vi "Doe_Julabo_Control_subVI_2.vi"(0 "Julabo CF41 VISA":refnum<visa-resource-name>="COM3", 1 "Data Cluster In":T1={"Current DoE"=[], "SSI 1 Flow Rate"=0.0, "SSI 2 Flow Rate"=0.0, "FLOM 1 Flow Rate"=0.0, "FLOM 2 Flow Rate"=0.0, "Pumps Running?"=FALSE, "Boolean 2"=FALSE, "Boolean 3"=FALSE, "Boolean 4"=FALSE, "At Equilibrium?"=FALSE, "Script Running?"=FALSE, "Current Script Iteration"=0.0, "Total Script Iterations"=0.0, "FLOM Pumps VISA"="COM2", "SSI 1 Pump VISA"="COM76", "SSI 2 Pump VISA"="COM74", "Huber Unistat VISA"="COM1", "SSI 3 Pump VISA"="COM76", "SSI 4 Pump VISA"="COM76", "SSI 4 Flow Rate"=0.0, "SSI 3 Flow Rate"=0.0, "Flow Meter 1 Rate "=0.0, "Flow Meter 2 Rate"=0.0, "Flow Meter 3 Rate"=0.0, "Flow Meter 4 Rate"=0.0, "SSI 1 Flow Setpoint"=0.0, "SSI 2 Flow Setpoint"=0.0, "SSI 3 Flow Setpoint"=0.0, "SSI 4 Flow Setpoint"=0.0, "Temperature Setpoint"=0.0, "Flow meter 3 COM"=17, "Flow meter 5 COM"=18, "Flow meter 4 COM"=19, "Flow meter 2 COM"=16, "Flow meter 1 COM"=15, "Unit"=enum."PSI", "Pressure COM"="COM6", "Julabo Setpoint"=0.0, "Julabo Control"=enum."Internal", "Overtemp"=50.0, "Subtemp"=-20.0, "HeatMax"=50, "CoolMax"=-100, "InternMax"=50.0, "InternMin"=0.0, "Upper Bandlimit"=100.0, "Lower Bandlimit"=0.0, "Julabo CF41 VISA"="COM3", "Xp (0.6K) Int"=0.6, "Tn (3s) Int"=3, "Tv (0s) Int"=0, "Dynamic (0: aperiodic) Int"=enum."aperiodic", "Xp (0.6K) Ext"=0.6, "Tn (3s) Ext"=3, "Tv (0s) Ext"=0, "XpU (0.6K) Ext"=0.6, "Julabo Serial Configuration"={"Baud Rate"=4800, "Parity"=2, "Data Bits"=7, "Stop Bits"=10, "Flow Control"=2}} {"Julabo Serial Configuration"."Flow Control" items=["None", "XON/XOFF", "RTS/CTS", "XON/XOFF & RTS/CTS", "DTR/DSR", "XON/XOFF & DTR/DSR"]; "Julabo Serial Configuration"."Stop Bits" items=["1.0"=10, "1.5"=15, "2.0"=20]; "Julabo Serial Configuration"."Data Bits" items=["7"=7, "8"=8]; "Julabo Serial Configuration"."Parity" items=["None", "Odd", "Even", "Mark", "Space"]; "Julabo Serial Configuration"."Baud Rate" items=["300"=300, "600"=600, "1200"=1200, "2400"=2400, "4800"=4800, "9600"=9600, "19200"=19200]; "XpU (0.6K) Ext" min=0.1 max=99.9; "Tv (0s) Ext" max=999; "Tn (3s) Ext" min=3 max=9999; "Xp (0.6K) Ext" min=0.1 max=99.9; "Tv (0s) Int" max=999; "Tn (3s) Int" min=3 max=9999; "Xp (0.6K) Int" min=0.1 max=99.9; "Lower Bandlimit" min=0.0 max=200.0; "Upper Bandlimit" min=0.0 max=200.0; "InternMin" format="%.2f"; "InternMax" format="%.2f"; "CoolMax" min=-100 max=0; "HeatMax" max=100; "Subtemp" format="%.2f"; "Overtemp" format="%.2f"; "Julabo Setpoint" format="%.2f"; "Current DoE" format="%0.3f"}, 2 "Case Selector":string, 3 "StartStop":bool) -> (4 "Data Cluster Out":T1={"Current DoE"=[], "SSI 1 Flow Rate"=0.0, "SSI 2 Flow Rate"=0.0, "FLOM 1 Flow Rate"=0.0, "FLOM 2 Flow Rate"=0.0, "Pumps Running?"=FALSE, "Boolean 2"=FALSE, "Boolean 3"=FALSE, "Boolean 4"=FALSE, "At Equilibrium?"=FALSE, "Script Running?"=FALSE, "Current Script Iteration"=0.0, "Total Script Iterations"=0.0, "FLOM Pumps VISA"="COM2", "SSI 1 Pump VISA"="COM76", "SSI 2 Pump VISA"="COM74", "Huber Unistat VISA"="COM1", "SSI 3 Pump VISA"="COM76", "SSI 4 Pump VISA"="COM76", "SSI 4 Flow Rate"=0.0, "SSI 3 Flow Rate"=0.0, "Flow Meter 1 Rate "=0.0, "Flow Meter 2 Rate"=0.0, "Flow Meter 3 Rate"=0.0, "Flow Meter 4 Rate"=0.0, "SSI 1 Flow Setpoint"=0.0, "SSI 2 Flow Setpoint"=0.0, "SSI 3 Flow Setpoint"=0.0, "SSI 4 Flow Setpoint"=0.0, "Temperature Setpoint"=0.0, "Flow meter 3 COM"=17, "Flow meter 5 COM"=18, "Flow meter 4 COM"=19, "Flow meter 2 COM"=16, "Flow meter 1 COM"=15, "Unit"=enum."PSI", "Pressure COM"="COM6", "Julabo Setpoint"=0.0, "Julabo Control"=enum."Internal", "Overtemp"=50.0, "Subtemp"=-20.0, "HeatMax"=50, "CoolMax"=-100, "InternMax"=50.0, "InternMin"=0.0, "Upper Bandlimit"=100.0, "Lower Bandlimit"=0.0, "Julabo CF41 VISA"="COM3", "Xp (0.6K) Int"=0.6, "Tn (3s) Int"=3, "Tv (0s) Int"=0, "Dynamic (0: aperiodic) Int"=enum."aperiodic", "Xp (0.6K) Ext"=0.6, "Tn (3s) Ext"=3, "Tv (0s) Ext"=0, "XpU (0.6K) Ext"=0.6, "Julabo Serial Configuration"={"Baud Rate"=4800, "Parity"=2, "Data Bits"=7, "Stop Bits"=10, "Flow Control"=2}} {"Julabo Serial Configuration"."Flow Control" items=["None", "XON/XOFF", "RTS/CTS", "XON/XOFF & RTS/CTS", "DTR/DSR", "XON/XOFF & DTR/DSR"]; "Julabo Serial Configuration"."Stop Bits" items=["1.0"=10, "1.5"=15, "2.0"=20]; "Julabo Serial Configuration"."Data Bits" items=["7"=7, "8"=8]; "Julabo Serial Configuration"."Parity" items=["None", "Odd", "Even", "Mark", "Space"]; "Julabo Serial Configuration"."Baud Rate" items=["300"=300, "600"=600, "1200"=1200, "2400"=2400, "4800"=4800, "9600"=9600, "19200"=19200]; "XpU (0.6K) Ext" min=0.1 max=99.9; "Tv (0s) Ext" max=999; "Tn (3s) Ext" min=3 max=9999; "Xp (0.6K) Ext" min=0.1 max=99.9; "Tv (0s) Int" max=999; "Tn (3s) Int" min=3 max=9999; "Xp (0.6K) Int" min=0.1 max=99.9; "Lower Bandlimit" min=0.0 max=200.0; "Upper Bandlimit" min=0.0 max=200.0; "InternMin" format="%.2f"; "InternMax" format="%.2f"; "CoolMax" min=-100 max=0; "HeatMax" max=100; "Subtemp" format="%.2f"; "Overtemp" format="%.2f"; "Julabo Setpoint" format="%.2f"; "Current DoE" format="%0.3f"}, 15 "error out 2":errorcluster caption="error out")   [LabVIEW 2015, in "JULABO DeviceDriver.lvlib"]
doc: "Advanced event triggered example"
uses:
  <instrlib>/JULABO DeviceDriver/JULABO DeviceDriver.lvlib
  --Controls and TypeDefs--/DoE_Control_Cluster.ctl
  <instrlib>/JULABO DeviceDriver/Examples/Julabo Serial Control.ctl
panel:
  in  "error in":errorcluster
  out "device error out":errorcluster
  in  "Setpointindex":enum16{"Setpoint 1", "Setpoint 2", "Setpoint 3"}(ring)
  in  "Registerkartenelement":T3(tab)
  # "Note: Julabo must be set to Set Temp - RS232\nfor commands to properly write to unit!!!!!"
  # "1. Select the COM-Port and adjust the serial\nconfiguration for your instrument\n2. Adjust the Read cycle\n3. Start the VI by pressing the \"Start\" -Button\n( Arrow button on the top-left corner)\n4. To stop the execution press the \"Stop\" button"
  # "Julabo"
  # "Limits"
  # "PID Control Parameters"
  # "Julabo"
  # "Limits"
  # "PID Control Parameters"
  # "Internal parameters"
  # "External parameters"
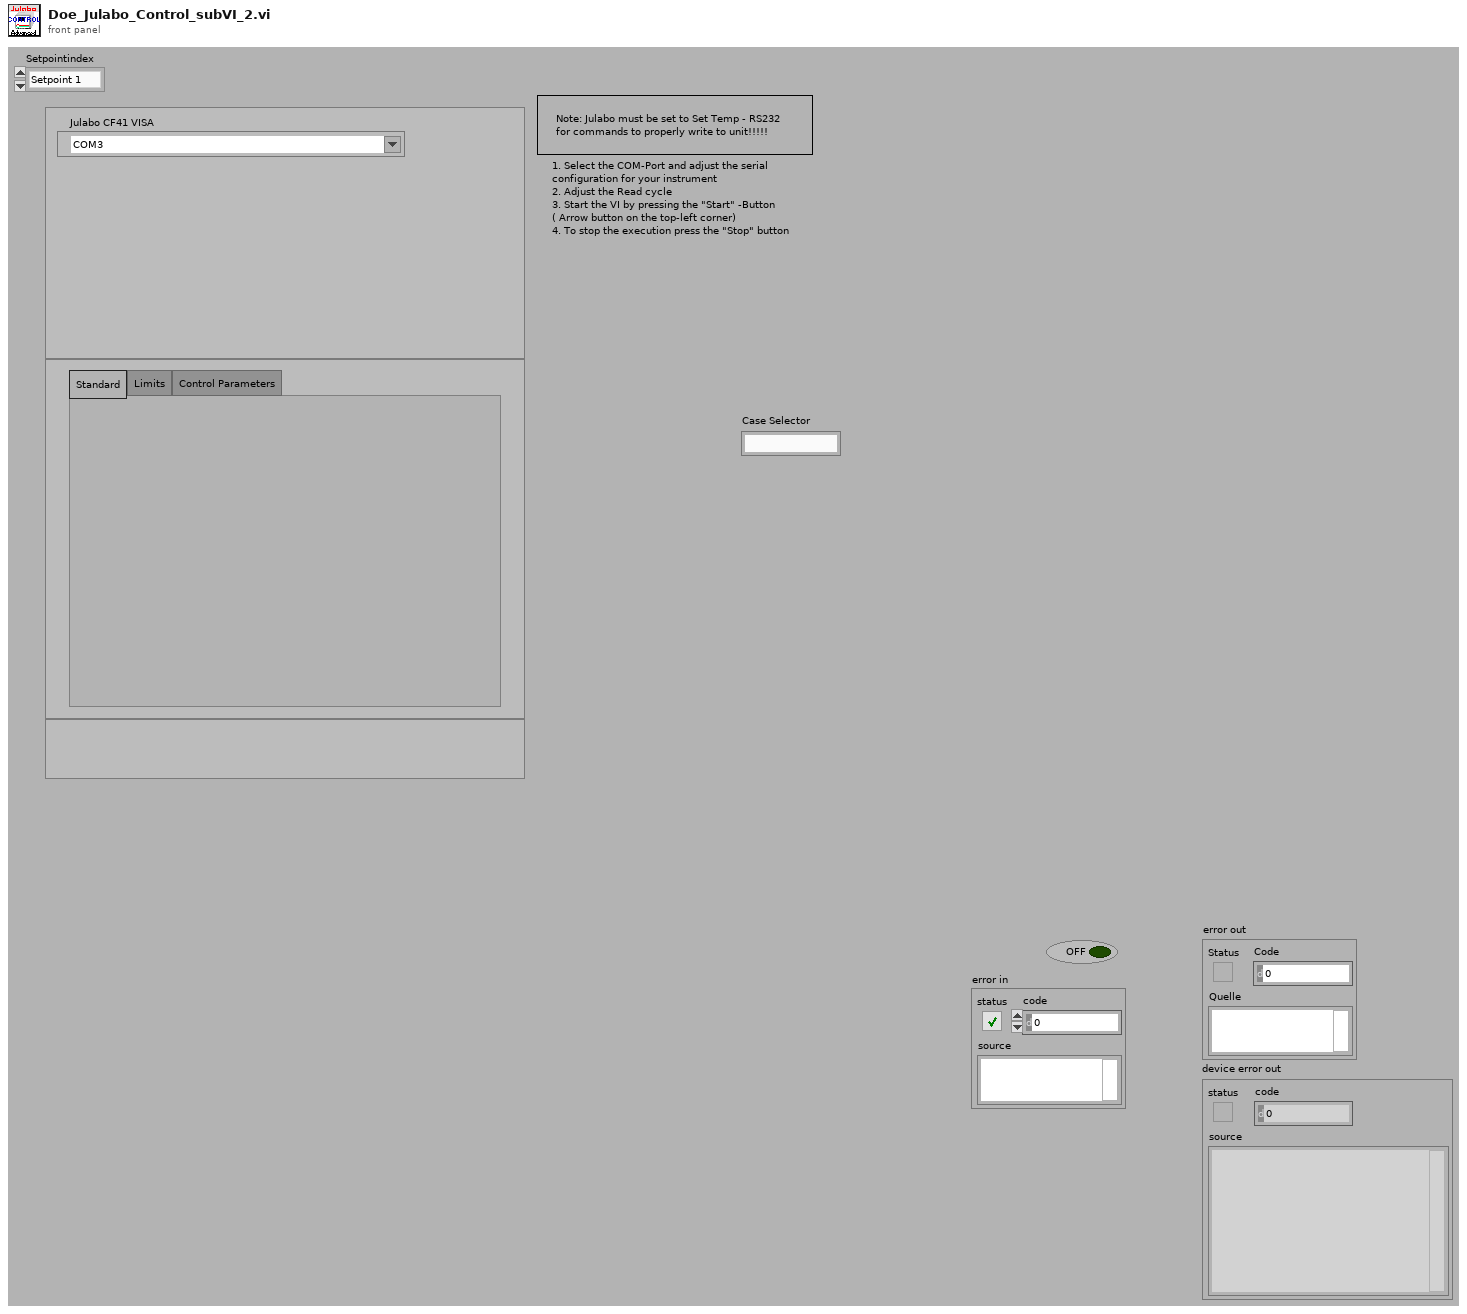
[diagram p1: front panel]
types:
  T1 = typedef "DoE_Control_Cluster.ctl" = cluster{"Current DoE":dbl[][], "SSI 1 Flow Rate":dbl, "SSI 2 Flow Rate":dbl, "FLOM 1 Flow Rate":dbl, "FLOM 2 Flow Rate":dbl, "Pumps Running?":bool, "Boolean 2":bool, "Boolean 3":bool, "Boolean 4":bool, "At Equilibrium?":bool, "Script Running?":bool, "Current Script Iteration":dbl, "Total Script Iterations":dbl, "FLOM Pumps VISA":refnum<visa-resource-name>, "SSI 1 Pump VISA":refnum<visa-resource-name>, "SSI 2 Pump VISA":refnum<visa-resource-name>, "Huber Unistat VISA":refnum<visa-resource-name>, "SSI 3 Pump VISA":refnum<visa-resource-name>, "SSI 4 Pump VISA":refnum<visa-resource-name>, "SSI 4 Flow Rate":dbl, "SSI 3 Flow Rate":dbl, "Flow Meter 1 Rate ":dbl, "Flow Meter 2 Rate":dbl, "Flow Meter 3 Rate":dbl, "Flow Meter 4 Rate":dbl, "SSI 1 Flow Setpoint":dbl, "SSI 2 Flow Setpoint":dbl, "SSI 3 Flow Setpoint":dbl, "SSI 4 Flow Setpoint":dbl, "Temperature Setpoint":dbl, "Flow meter 3 COM":u16, "Flow meter 5 COM":u16, "Flow meter 4 COM":u16, "Flow meter 2 COM":u16, "Flow meter 1 COM":u16, "Unit":enum16{"PSI", "Bar", "cm H2O", "ft H2O", "hectoPascal", "in Hg", "in H2O", "kiloPascal", "milliBar", "mmHg", "MegaPascal", "Numeric Pressure"}, "Pressure COM":refnum<visa-resource-name>, "Julabo Setpoint":dbl, "Julabo Control":enum16{"Internal", "External"}, "Overtemp":dbl, "Subtemp":dbl, "HeatMax":u8, "CoolMax":i8, "InternMax":dbl, "InternMin":dbl, "Upper Bandlimit":dbl, "Lower Bandlimit":dbl, "Julabo CF41 VISA":refnum<visa-resource-name>, "Xp (0.6K) Int":dbl, "Tn (3s) Int":u16, "Tv (0s) Int":u16, "Dynamic (0: aperiodic) Int":enum16{"aperiodic", "standard"}, "Xp (0.6K) Ext":dbl, "Tn (3s) Ext":u16, "Tv (0s) Ext":u16, "XpU (0.6K) Ext":dbl, "Julabo Serial Configuration":T2}
  T2 = typedef "Julabo Serial Control.ctl" = cluster{"Baud Rate":u32, "Parity":u16, "Data Bits":u16, "Stop Bits":u16, "Flow Control":u16}
  T3 = enum32{"Standard", "Limits", "Control Parameters"}
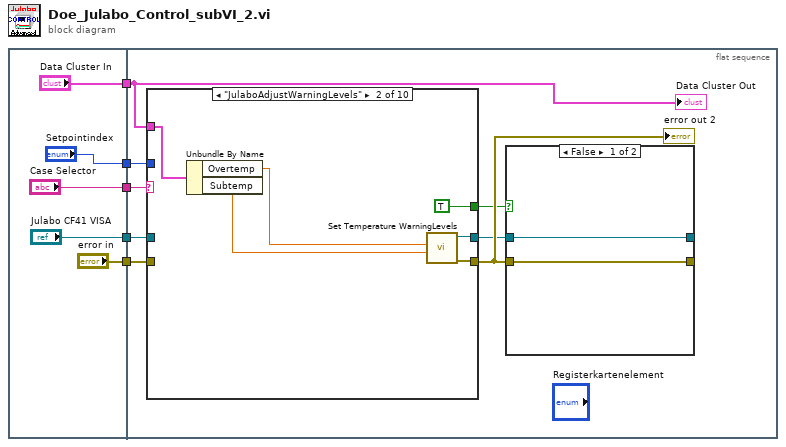
[diagram p0: block diagram]
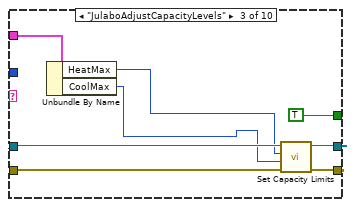
[diagram p3: hidden frame]
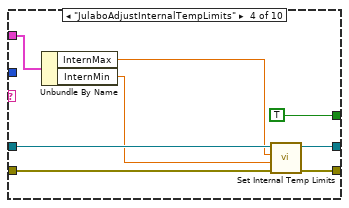
[diagram p4: hidden frame]
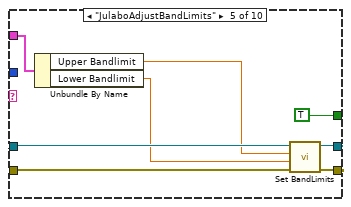
[diagram p5: hidden frame]
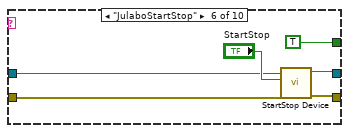
[diagram p6: hidden frame]
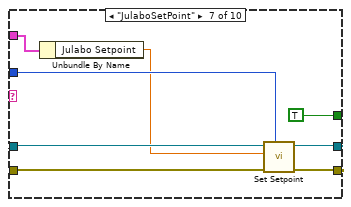
[diagram p7: hidden frame]
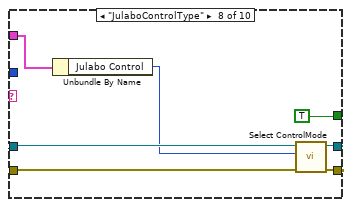
[diagram p8: hidden frame]
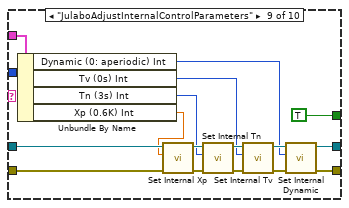
[diagram p9: hidden frame]
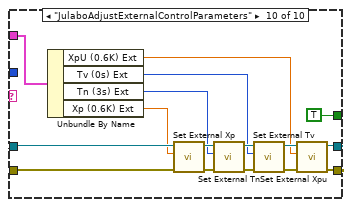
[diagram p10: hidden frame]
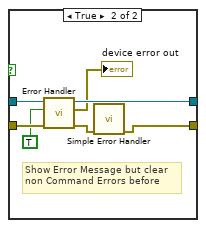
[diagram p11: hidden frame]
diagram:
  n1 = flat-sequence {
    tunnel: ["Setpointindex"] -> w5
    tunnel: ["Julabo CF41 VISA"] -> w4
    tunnel: ["error in"] -> w3
    tunnel: ["Case Selector"] -> w2
    tunnel: ["Data Cluster In"] -> w1
    tunnel: w5 -> [w13]
    tunnel: w4 -> [w14]
    tunnel: w3 -> [w15]
    tunnel: w2 -> [w12]
    tunnel: w1 -> [w11]
    frame #0 {
    }
    frame #1 {
      n2 = case shown="\"JulaboAdjustWarningLevels\"" w12 {
        tunnel: w15 -> [w20 _ w34 w42 w50 w55 w64 w71 w81 w97]
        tunnel: w14 -> [w19 _ w33 w41 w49 w54 w62 w70 w80 w96]
        tunnel: [w19 w26 w31 w39 w47 w53 w60 w68 w78 w94] -> w17
        tunnel: [w20 w25 w30 w40 w46 w52 w61 w69 w79 w95] -> w18
        tunnel: [_ TRUE TRUE TRUE TRUE TRUE TRUE TRUE TRUE TRUE] -> w16
        tunnel: w13 -> [_ _ _ _ _ _ w63 _ _ _]
        tunnel: w11 -> [_ w23 w29 w37 w45 _ w58 w66 w76 w92]
        frame Default {
        }
        frame "JulaboAdjustWarningLevels" {
          n3 = Unbundle By Name(w23) -> ("Overtemp"=w22:dbl, "Subtemp"=w21:dbl)
          n4 = call <instrlib>:"Set Temperature WarningLevels.vi"("Subtemp (-20.00°C)"=w21, "Overtemp (50.00°C)"=w22) -> ("error out"=w25:errorcluster, "VISA resource name out"=w26:refnum<visa-resource-name>)  [unwired: 8 in]
        }
        frame "JulaboAdjustCapacityLevels" {
          n5 = Unbundle By Name(w29) -> ("HeatMax"=w27:u8, "CoolMax"=w28:i8)
          n6 = call <instrlib>:"Set Capacity Limits.vi"("error in (no error)"=w34, "Maximum cooling capacity(-100%)"=w28, "Maximum heating capacity(100%)"=w27, "VISA resource name"=w33) -> ("error out"=w30:errorcluster, "VISA resource name out"=w31:refnum<visa-resource-name>)  [unwired: 6 in]
        }
        frame "JulaboAdjustInternalTempLimits" {
          n7 = Unbundle By Name(w37) -> ("InternMax"=w36:dbl, "InternMin"=w35:dbl)
          n8 = call <instrlib>:"Set Internal Temp Limits.vi"("error in (no error)"=w42, "InternMin (-20.00 °C)"=w35, "InternMax (50.00 °C)"=w36, "VISA resource name"=w41) -> ("error out"=w40:errorcluster, "VISA resource name out"=w39:refnum<visa-resource-name>)  [unwired: 6 in]
        }
        frame "JulaboAdjustBandLimits" {
          n9 = Unbundle By Name(w45) -> ("Upper Bandlimit"=w44:dbl, "Lower Bandlimit"=w43:dbl)
          n10 = call <instrlib>:"Set BandLimits.vi"("error in (no error)"=w50, "Lower Bandlimit (200K)"=w43, "Upper Bandlimit (200K)"=w44, "VISA resource name"=w49) -> ("error out"=w46:errorcluster, "VISA resource name out"=w47:refnum<visa-resource-name>)  [unwired: 6 in]
        }
        frame "JulaboStartStop" {
          n11 = call <instrlib>:"StartStop Device.vi"("error in (no error)"=w55, "Start/Stop (f:Stop)"="StartStop", "VISA resource name"=w54) -> ("error out"=w52:errorcluster, "VISA resource name out"=w53:refnum<visa-resource-name>)  [unwired: 7 in]
        }
        frame "JulaboSetPoint" {
          n12 = Unbundle By Name(w58) -> ("Julabo Setpoint"=w57:dbl)
          n13 = call <instrlib>:"Set Setpoint.vi"("Setpointindex (Setpoint1: Default)"=w63, "error in (no error)"=w64, "newSetpoint (20.00°C)"=w57, "VISA resource name"=w62) -> ("error out"=w61:errorcluster, "VISA resource name out"=w60:refnum<visa-resource-name>)  [unwired: 6 in]
        }
        frame "JulaboControlType" {
          n14 = Unbundle By Name(w66) -> ("Julabo Control"=w65:enum16{"Internal", "External"})
          n15 = call <instrlib>:"Select ControlMode.vi"("error in (no error)"=w71, "Control (0: Internal)"=w65, "VISA resource name"=w70) -> ("error out"=w69:errorcluster, "VISA resource name out"=w68:refnum<visa-resource-name>)  [unwired: 7 in]
        }
        frame "JulaboAdjustInternalControlParameters" {
          n16 = Unbundle By Name(w76) -> ("Dynamic (0: aperiodic) Int"=w72:enum16{"aperiodic", "standard"}, "Tv (0s) Int"=w73:u16, "Tn (3s) Int"=w74:u16, "Xp (0.6K) Int"=w75:dbl)
          n17 = call <instrlib>:"Set Internal Xp.vi"("error in (no error)"=w81, "Xp (0.6K)"=w75, "VISA resource name"=w80) -> ("error out"=w84:errorcluster, "VISA resource name out"=w85:refnum<visa-resource-name>)  [unwired: 7 in]
          n18 = call <instrlib>:"Set Internal Tn.vi"("error in (no error)"=w84, "Tn (3s)"=w74, "VISA resource name"=w85) -> ("error out"=w82:errorcluster, "VISA resource name out"=w83:refnum<visa-resource-name>)  [unwired: 7 in]
          n19 = call <instrlib>:"Set Internal Tv.vi"("error in (no error)"=w82, "Tv (0s)"=w73, "VISA resource name"=w83) -> ("error out"=w87:errorcluster, "VISA resource name out"=w86:refnum<visa-resource-name>)  [unwired: 7 in]
          n20 = call <instrlib>:"Set Internal Dynamic.vi"("error in (no error)"=w87, "Dynamic (0: aperiodic)"=w72, "VISA resource name"=w86) -> ("error out"=w79:errorcluster, "VISA resource name out"=w78:refnum<visa-resource-name>)  [unwired: 7 in]
        }
        frame "JulaboAdjustExternalControlParameters" {
          n21 = Unbundle By Name(w92) -> ("XpU (0.6K) Ext"=w88:dbl, "Tv (0s) Ext"=w89:u16, "Tn (3s) Ext"=w90:u16, "Xp (0.6K) Ext"=w91:dbl)
          n22 = call <instrlib>:"Set External Xp.vi"("error in (no error)"=w97, "Xp (0.6K)"=w91, "VISA resource name"=w96) -> ("error out"=w100:errorcluster, "VISA resource name out"=w101:refnum<visa-resource-name>)  [unwired: 7 in]
          n23 = call <instrlib>:"Set External Tn.vi"("error in (no error)"=w100, "Tn (3s)"=w90, "VISA resource name"=w101) -> ("error out"=w98:errorcluster, "VISA resource name out"=w99:refnum<visa-resource-name>)  [unwired: 7 in]
          n24 = call <instrlib>:"Set External Tv.vi"("error in (no error)"=w98, "Tv (0s)"=w89, "VISA resource name"=w99) -> ("error out"=w103:errorcluster, "VISA resource name out"=w102:refnum<visa-resource-name>)  [unwired: 7 in]
          n25 = call <instrlib>:"Set External Xpu.vi"("error in (no error)"=w103, "XpU (0.6K)"=w88, "VISA resource name"=w102) -> ("error out"=w95:errorcluster, "VISA resource name out"=w94:refnum<visa-resource-name>)  [unwired: 7 in]
        }
      }
      "error out 2" <- w18
      n26 = case shown="False" w16 {
        tunnel: w17 -> [w105 w110]
        tunnel: [w105 w108] -> _
        tunnel: w18 -> [w104 w111]
        tunnel: [w104 w112] -> _
        frame False {
        }
        frame True {
          # "Show Error Message but clear\nnon Command Errors before"
          n27 = call <instrlib>:"Error Handler.vi"("error in (no error)"=w111, "ClearDeviceError (false)"=TRUE, "VISA resource name"=w110) -> ("error out"=w109:errorcluster, "device error out"=→"device error out":errorcluster, "VISA resource name out"=w108:refnum<visa-resource-name>)  [unwired: 5 in, 1 out]
          n28 = call <vilib>:"Simple Error Handler.vi"("error in (no error)"=w109) -> ("error out"=w112:errorcluster)  [unwired: 4 in, 4 out]
        }
      }
      "Data Cluster Out" <- w11
    }
  }
